vi "hReadChannels-UandP-2013.bak.vi"(0 "FPGA VI Reference In":refnum<k20>, 1 "SavGol side points":i32=10, 3 "Use Voltage or Power for AO?":bool, 4 "order polynomial":i32=2, 5 "Nsamples":u32=10000, 6 "error in":errorcluster, 8 "output cluster":T3, 9 "calculation settings":i32(slide) scale=0.0..3.0, 10 "variables cluster":T2, 11 "No. Of Samples to average":i32=10) -> (2 "Fehler":bool, 13 "AdjustedArray":sgl[][](array[numeric]), 18 "single channel voltage array":dbl[](array[numeric]), 19 "real time P_rad array":dbl[](array[numeric]), 20 "FPGA VI Reference Out":refnum<k20>, 22 "PowerArray":sgl[][](array[numeric]), 25 "RawArray":sgl[][](array[numeric]), 26 "error out":errorcluster)   [LabVIEW 2014]
doc: "startet das einlesen und führt dies bis n Samples aus\nHier mit FIFO und IRQ."
uses:
  <vilib>/Utility/error.llb/Error Cluster From Error Code.vi
  <vilib>/rvi/errors/niLvFpgaAdjustHostInterfaceError.vi
  <vilib>/RVI Host/nirviSupport.llb/nirviErrorClusterFromErrorCode.vi
  <vilib>/rvi/interface/nirviReadWriteControl/nirviReadWriteControl.xnode
  FPGA Bitfiles/W7XBolo2017_FPGATarget_fmain2014_DACRangeVoltage.lvbitx
  f_main_2014.vi
  <vilib>/rvi/interface/nirviMethod/nirviMethod.xnode
  NiFpgaLv.dll
  <vilib>/rvi/interface/nirviMethod/StockFPGA_InlinedMethodWaitForMultipleIRQ.vi
  <vilib>/FPGAPlugInAG/PCI-7813R/niLvFpga_WaitOnIrq_PCI-7813R.vi
  <vilib>/FPGAPlugInAG/PCI-7813R/niLvFpga_AcknowledgeIrq_PCI-7813R.vi
  <vilib>/FPGAPlugInAG/PCI-7813R/niLvFpga_ReadFifo_PCI-7813R.vi
  <vilib>/rvi/errors/niLvFpgaMergeErrorWithErrorCode.vi
panel:
  in  "Tab Control":T1(tab)
  out "16bit integer voltage sample":i16[](array[numeric])
  out "RTPRad voltage factor":dbl
  out "Timed Out":bool
  out "STOP?":bool
  out "Elements Remaining":u32
  out "single channel voltage":sgl
  out "single channel voltage * factor":dbl
  out "empty sample array":dbl[](array[numeric])
  out "Nsamples array":i64[](array[numeric])
  out "sample":i32
  out "new level of override":i32
  out "sate":string
  out "last U sample":sgl[](array[numeric])
  out "current P_rad [MW]":dbl
  out "rt prad average array":dbl[][](array[numeric])
  out "elec. channel selected":i64
  out "element of channel\nand sample":sgl
  out "column":i32
  out "channel index":i32
  out "av/f_OT*volume/k_bolo/V_cam":dbl
  out "average":dbl
  out "sum":dbl
  out "av/f_OT*volume":dbl
  out "average/f_OT":sgl
  out "av/f_OT*volume/k_bolo":dbl
  in  "magic number":dbl=1.0
  out "current power":sgl[](array[numeric])
  out "prad av array":dbl[](array[numeric])
  out "index status":bool
  out "dU/dt":sgl[](array[numeric])
  out "channel number":i64
  out "RawScal":dbl[](array[numeric])
  out "Scale(mV)":sgl[](array[numeric])
  out "SumScal":dbl[](array[numeric])
  out "Tau/dt":dbl[](array[numeric])
  out "F_ch":dbl[](array[numeric])
  out "tau_fact":dbl[](array[numeric])
  out "kbolott_and_volume":dbl[][](array[numeric])
  out "samples to exclude":u32
  out "single channel number":i64
  out "channelNumber":i32
  out "channelSelection":i64[][](array[numeric])
  out "tau_M":dbl[](array[numeric])
  out "Offsets":dbl[](array[numeric])
  out "SampleTime":sgl
  out "voltage factor":dbl
  out "Scale(mV) transf.":sgl[](array[numeric])
  out "V_cam":dbl
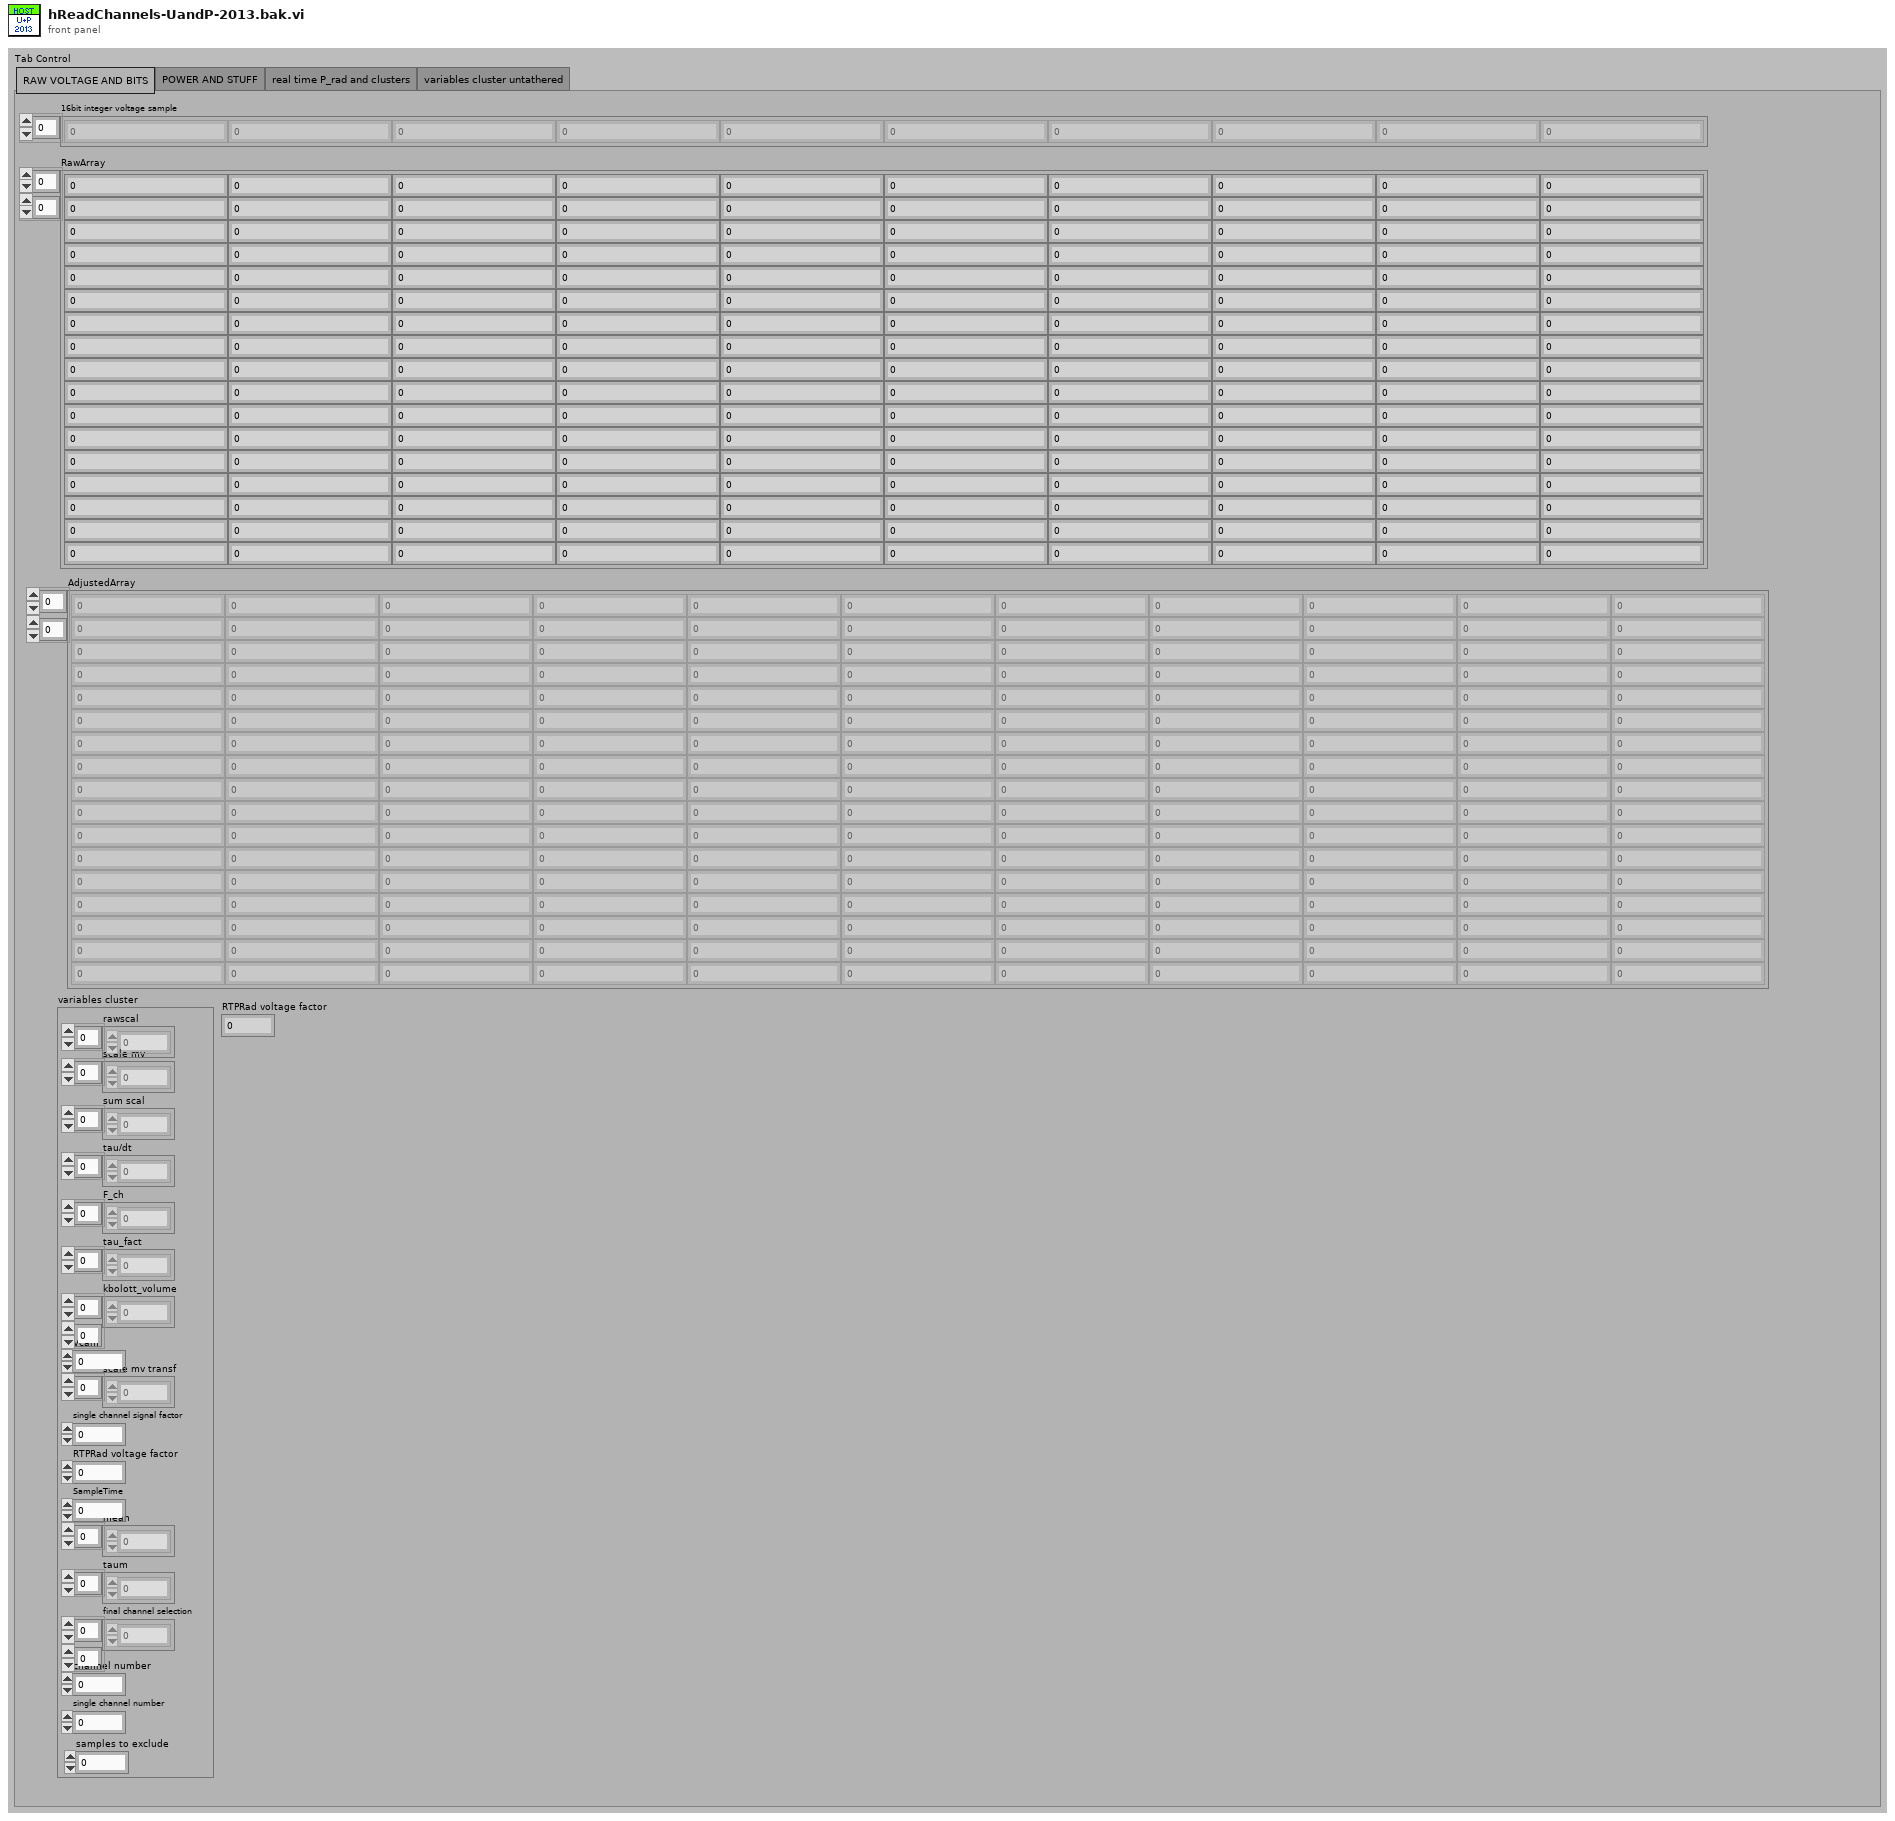
[diagram p1: front panel]
types:
  T1 = enum32{"RAW VOLTAGE AND BITS", "POWER AND STUFF", "real time P_rad and clusters", "variables cluster untathered"}
  T2 = cluster{"rawscal":dbl[], "scale mv":sgl[], "sum scal":dbl[], "tau/dt":dbl[], "F_ch":dbl[], "tau_fact":dbl[], "kbolott_volume":dbl[][], "Vcam":dbl, "scale mv transf":sgl[], "single channel signal factor":dbl, "RTPRad voltage factor":dbl, "SampleTime":sgl, "mean":dbl[], "taum":dbl[], "final channel selection":i64[][], "channel number":i32, "single channel number":i64, "samples to exclude":u32}
  T3 = cluster{"real time P_rad":refnum<vi>, "real time P_rad array":refnum<vi>, "single channel voltage":refnum<vi>, "single channel voltage array":refnum<vi>}
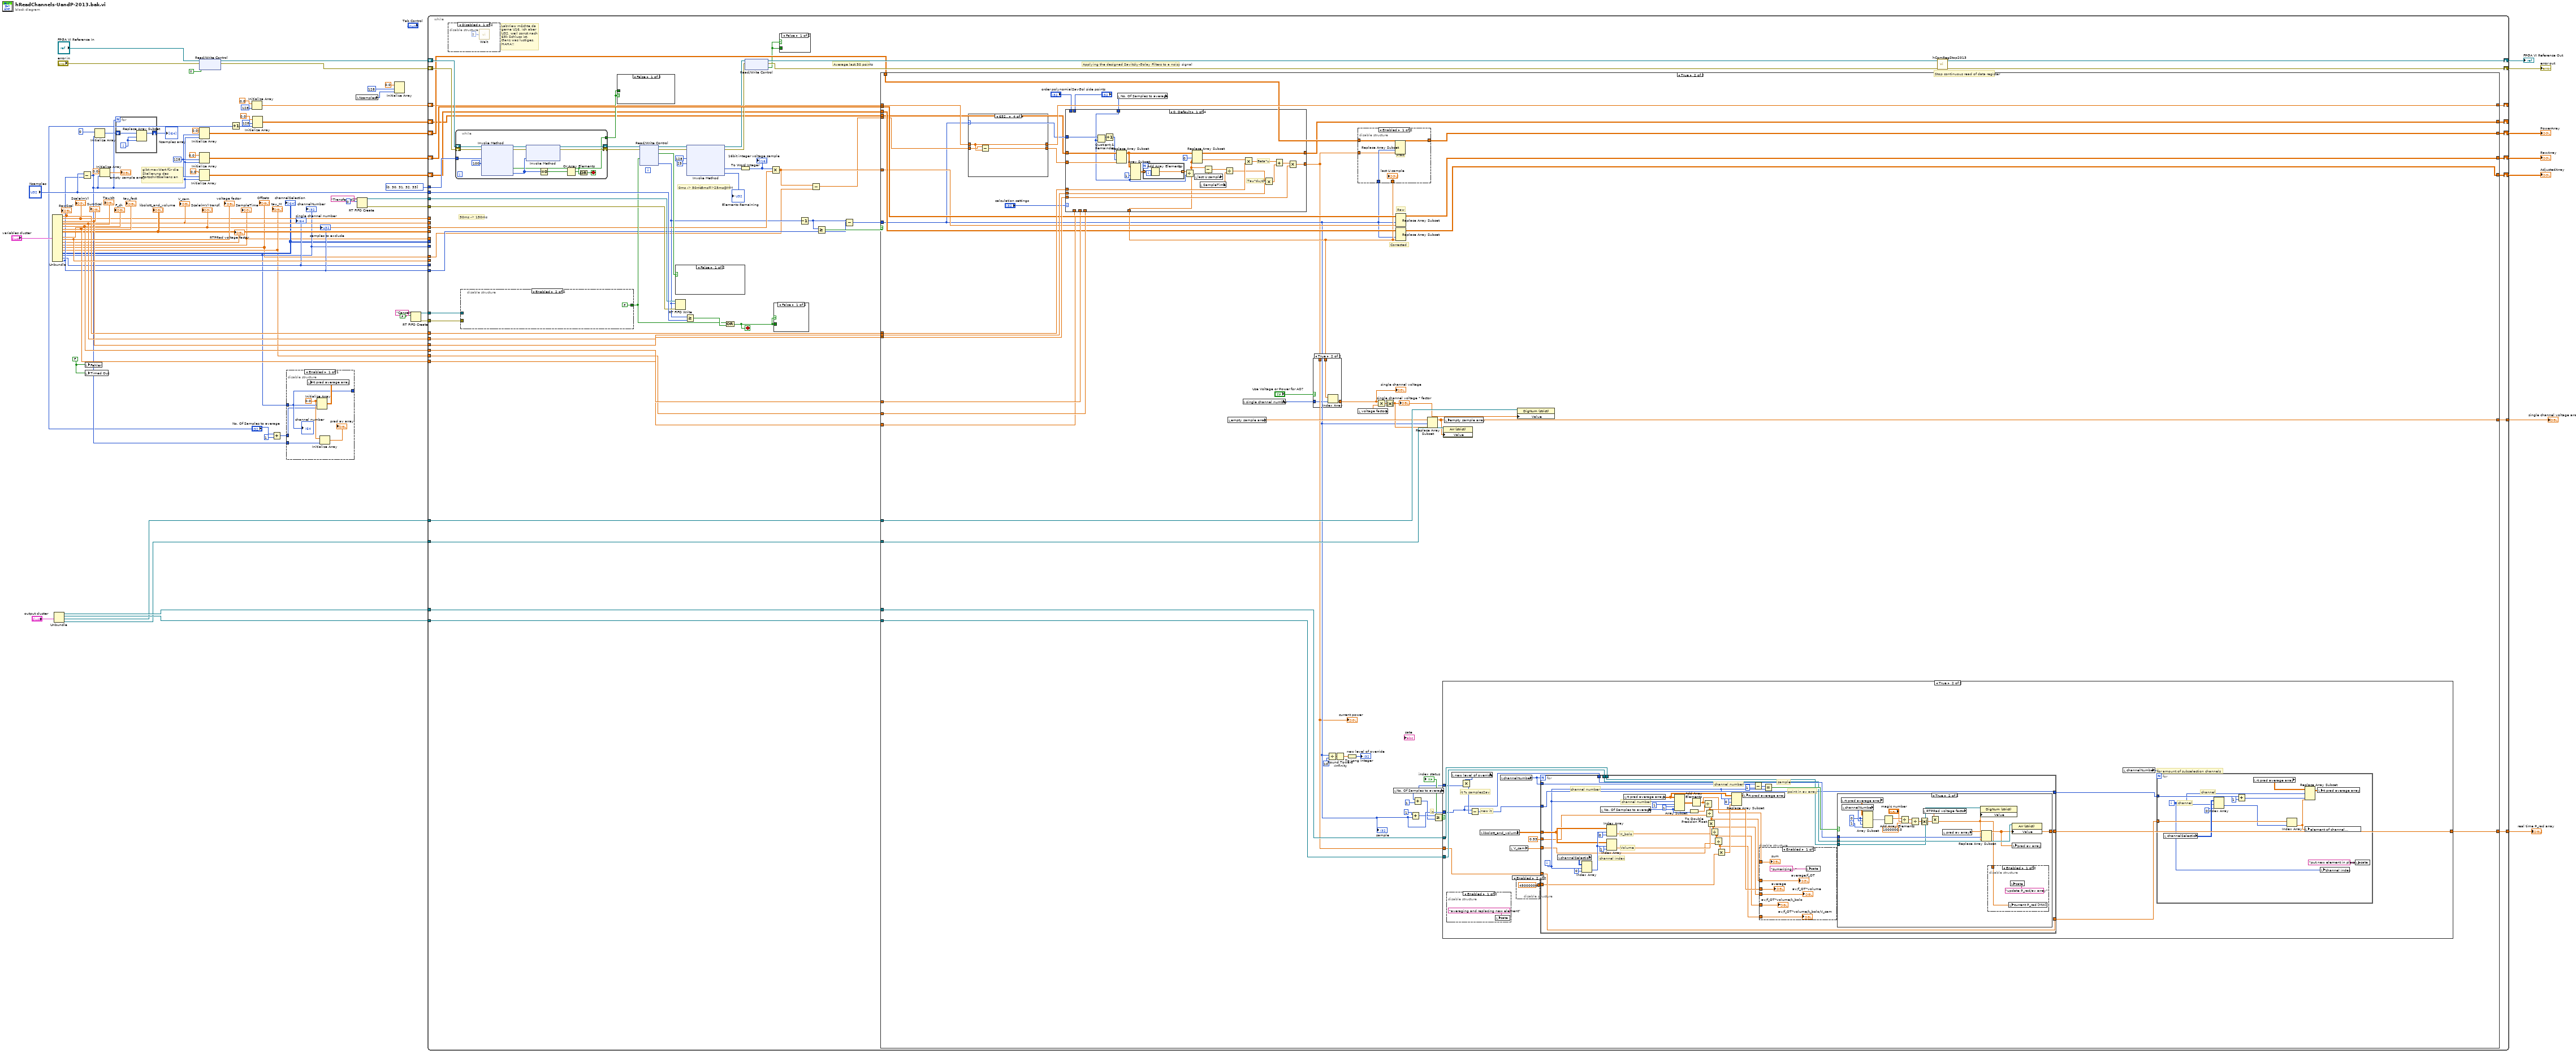
[diagram p0: block diagram]
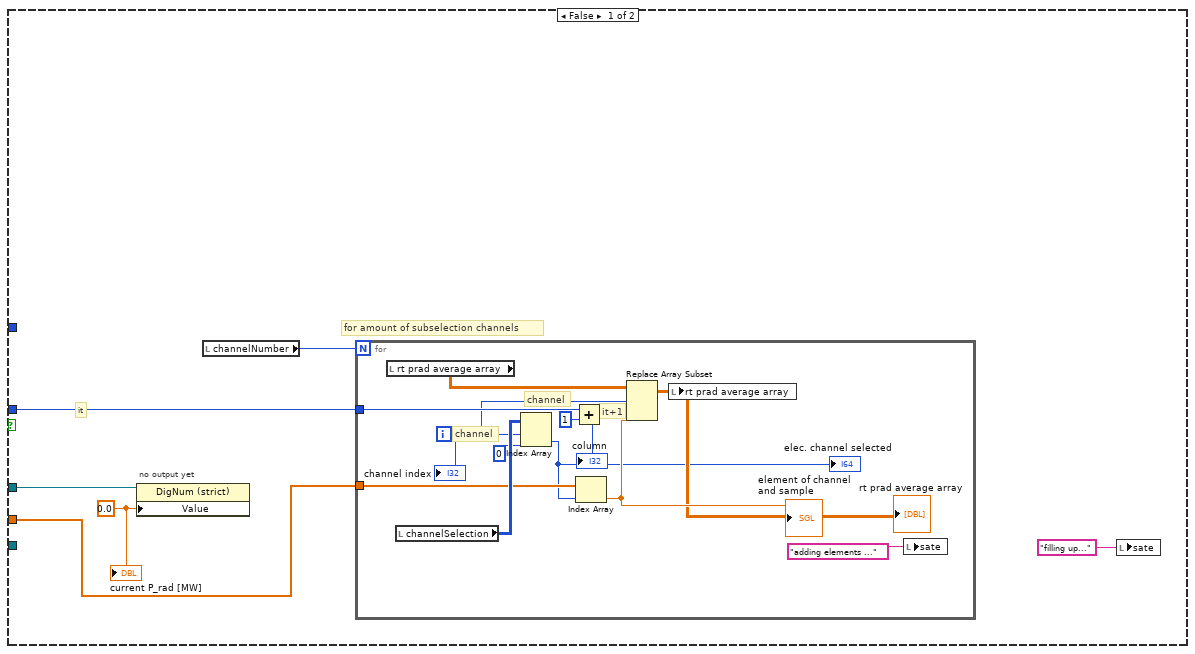
[diagram p3: hidden frame]
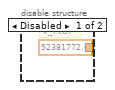
[diagram p4: hidden frame]
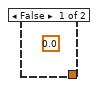
[diagram p7: hidden frame]
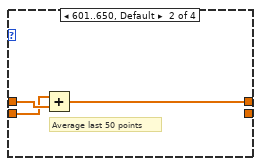
[diagram p10: hidden frame]
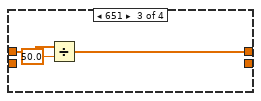
[diagram p11: hidden frame]
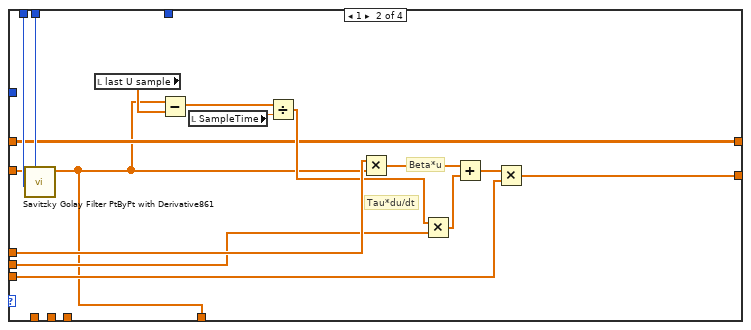
[diagram p12: hidden frame]
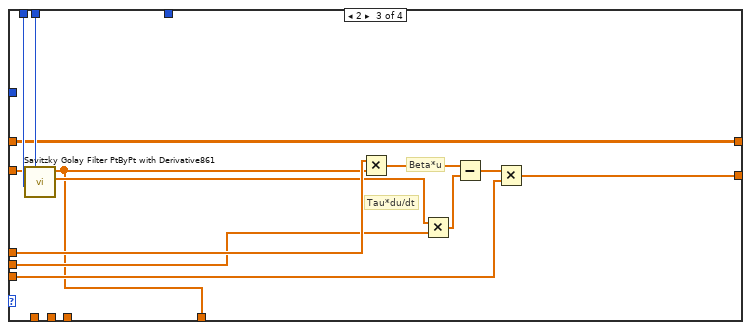
[diagram p13: hidden frame]
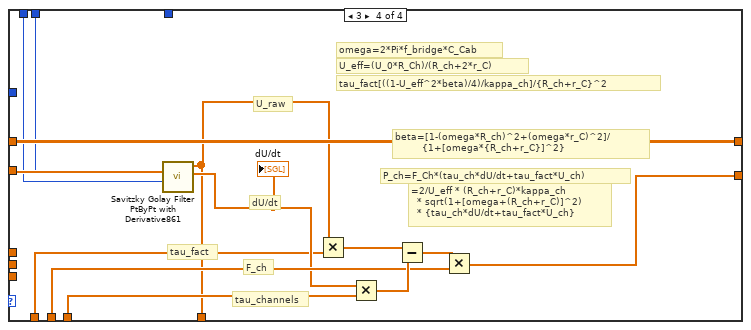
[diagram p14: hidden frame]
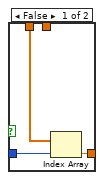
[diagram p15: hidden frame]
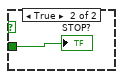
[diagram p17: hidden frame]
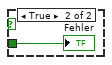
[diagram p18: hidden frame]
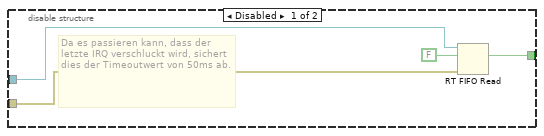
[diagram p19: hidden frame]
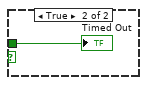
[diagram p20: hidden frame]
diagram:
  w44 = FALSE
  w19 = 128 ("dimension size")
  # "Stop continuous read of data register"
  # "gibt maxWert für die Skalierung des Fortschrittbalkens an"
  n1 = Unbundle("variables cluster") -> ("rawscal"=w35:dbl[], "scale mv"=w30:sgl[], "sum scal"=w36:dbl[], "tau/dt"=w34:dbl[], "F_ch"=w33:dbl[], "tau_fact"=w32:dbl[], "kbolott_volume"=w31:dbl[][], "Vcam"=w28:dbl, "scale mv transf"=w29:sgl[], "single channel signal factor"=w37:dbl, "RTPRad voltage factor"=→"RTPRad voltage factor":dbl, "SampleTime"=w8:sgl, "mean"=w9:dbl[], "taum"=w10:dbl[], "final channel selection"=w11:i64[][], "channel number"=w12:i32, "single channel number"=w13:i64, "samples to exclude"=w14:u32)
  "RawScal" <- w35
  "Scale(mV)" <- w30
  "SumScal" <- w36
  "Tau/dt" <- w34
  "F_ch" <- w33
  "tau_fact" <- w32
  "kbolott_and_volume" <- w31
  "V_cam" <- w28
  "Scale(mV) transf." <- w29
  "voltage factor" <- w37
  "SampleTime" <- w8
  "Offsets" <- w9
  "tau_M" <- w10
  "channelSelection" <- w11
  "channelNumber" <- w12
  "single channel number" <- w13
  "samples to exclude" <- w14
  n2 = Unbundle("output cluster") -> ("real time P_rad"=w39:refnum<vi>, "real time P_rad array"=w38:refnum<vi>, "single channel voltage"=w24:refnum<vi>, "single channel voltage array"=w23:refnum<vi>)
  n3 = Subtract(x="Nsamples", y=w14) -> (x-y=w18:u32)
  n4 = local write "Fehler"(w44) -> ()
  n5 = local write "Timed Out"(w44) -> ()
  n6 = Initialize Array(i64 0 ("element"), w18) -> (w46:i64[])
  n7 = Initialize Array(0.0 ("element"), w18) -> (→"empty sample array":dbl[])
  n8 = for {
    N: w18 -> [_]
    shift-right: [w76] -> w45
    shift-left: w46 -> [w78]
    i -> [w77]
    n9 = Replace Array Subset(array=w78, new element=w77, index=w77) -> (w76:i64[])
  }
  "Nsamples array" <- w45
  n10 = Initialize Array(sgl 0.0 ("element"), w19, w18) -> (w17:sgl[][])
  n11 = xnode "Read/Write Control"("FPGA VI Reference In"="FPGA VI Reference In", "error in"="error in", "ADCRead"=TRUE) -> ("FPGA VI Reference Out"=w57:refnum<k20>, "error out"=w56:errorcluster)
  n12 = Initialize Array(sgl 0.0 ("i"), w19, w18) -> (w66:sgl[][])
  n13 = Initialize Array(sgl 0.0, w19, w18) -> (w75:sgl[][])
  n14 = Increment(x="No. Of Samples to average") -> (x+1=w1:i32)
  n15 = Initialize Array(sgl 0.0 ("element"), 128 ("dimension size")) -> (w52:sgl[])
  n16 = Initialize Array(sgl 0.0 ("element"), 128 ("dimension size"), w1) -> (w3:sgl[][])
  n17 = Add(x="No. Of Samples to average", y=1) -> (x+y=w26:i32)
  n18 = disable-structure shown="Enabled" {
    disable-tunnel: w12 -> [w83]
    disable-tunnel: [w83] -> _
    disable-tunnel: w26 -> [w79]
    disable-tunnel: w18 -> [w80]
    frame Enabled {
      w82 = 0.0 ("element")
      n19 = Initialize Array(w82, w83, w79) -> (w84:dbl[][])
      n20 = local write "rt prad average array"(w84) -> ()
      n21 = Initialize Array(w82, w80) -> (→"prad av array":dbl[])
      "channel number" <- w83
    }
  }
  n22 = local read "Nsamples"() -> (w41:u32)
  n23 = RT FIFO Create(0:"Transferred1" ("name (unnamed)"), 1:u32 0) -> (8:w72:refnum<k33>, 11:w71:errorcluster)  [unwired: 2 in, 5 out]
  n24 = Initialize Array(sgl 0.0 ("element"), 128 ("dimension size"), w41) -> ()  [unwired: 1 out]
  n25 = RT FIFO Create(0:"Cancel" ("name (unnamed)"), 1:FALSE) -> (8:w69:refnum<k33>, 11:w68:errorcluster)  [unwired: 2 in, 5 out]
  n26 = while {
    tunnel: "Nsamples" -> [w137]
    shift-right: [w105] -> w15
    shift-left: w75 -> [w126]
    shift-right: [w138] -> w65
    shift-left: w57 -> [w141]
    shift-right: [w139] -> w64
    shift-left: w56 -> [w140]
    tunnel: w72 -> [w136]
    tunnel: w71 -> [w135]
    tunnel: w69 -> [w133]
    tunnel: w68 -> [w132]
    shift-right: [w130] -> w60
    shift-left: w66 -> [w131]
    tunnel: w29 -> [w125]
    tunnel: w34 -> [w122]
    tunnel: w36 -> [w124]
    tunnel: w35 -> [w123]
    shift-right: [w115] -> _
    shift-left: w52 -> [w91]
    tunnel: i32[] [0, 30, 31, 32, 33] -> [w110]
    tunnel: w23 -> [w107]
    tunnel: w24 -> [w106]
    tunnel: w13 -> [_]
    tunnel: w37 -> [_]
    tunnel: w9 -> [w87]
    tunnel: w14 -> [w88]
    tunnel: w39 -> [w102]
    tunnel: w38 -> [w97]
    tunnel: w33 -> [w101]
    tunnel: w32 -> [w100]
    tunnel: w30 -> [_]
    tunnel: w31 -> [_]
    tunnel: w8 -> [_]
    tunnel: w10 -> [w99]
    tunnel: w11 -> [_]
    tunnel: w12 -> [_]
    tunnel: w28 -> [_]
    tunnel: [w96] -> w22
    tunnel: [w95] -> w21
    shift-right: [w93] -> w16
    shift-left: w17 -> [w94]
    shift-right: [w85] -> _
    shift-left: w3 -> [w86]
    stop <- w111 stop-if-true
    # "Average last 50 points"
    # "Applying the designed Savitzky-Golay Filters to a noisy signal"
    # "LabView möchte da gerne U16, ich aber U32, weil sonst nach 65k Schluss ist. \nGanz was lustiges, HAHA!!"
    # "5ms=>25ms@MM"
    # "0ms -> 50ms"
    # "50ms -> 150ms"
    n27 = disable-structure shown="Disabled" {
      frame Disabled {
        n28 = call "Wait"("Count(uSec)"=u32 5) -> ()  [unwired: 1 out]
      }
      frame Enabled {
      }
    }
    n29 = while {
      tunnel: [w404] -> w114
      shift-right: [w406] -> w108
      shift-left: w141 -> [w413]
      shift-right: [w405] -> w109
      shift-left: w140 -> [w412]
      tunnel: w110 -> [w410]
      stop <- w403 stop-if-true
      n30 = xnode "Invoke Method"("FPGA VI Reference In"=w413, "error in"=w412, "IRQ Number(s)"=w410, "Timeout (ms)"=100) -> ("FPGA VI Reference Out"=w407:refnum<k20>, "error out"=w408:errorcluster, "Timed Out"=w404:bool, "IRQ(s) Asserted"=w409:i32[])
      n31 = xnode "Invoke Method"("FPGA VI Reference In"=w407, "error in"=w408, "IRQ Number(s)"=w409) -> ("FPGA VI Reference Out"=w406:refnum<k20>, "error out"=w405:errorcluster)
      n32 = Equal To 0?(x=w409) -> (x = 0?=w402:bool[])
      n33 = Or Array Elements(Boolean array=w402) -> (logical OR=w401:bool)
      n34 = Or(x=w401, y=w404) -> (x .or. y?=w403:bool)
    }
    n35 = disable-structure shown="Enabled" {
      disable-tunnel: [w419 FALSE] -> w134
      disable-tunnel: w133 -> [w418 _]
      disable-tunnel: w132 -> [w417 _]
      frame Disabled {
        # "Da es passieren kann, dass der letzte IRQ verschluckt wird, sichert dies der Timeoutwert von 50ms ab."
        n36 = RT FIFO Read(0:w418, 1:FALSE ("element"), 3:w417) -> (9:w419:bool)  [unwired: 5 out]
      }
      frame Enabled {
      }
    }
    n37 = case shown="False" w114 {
      tunnel: w114 -> [_ w421]
      frame False {
      }
      frame True {
        "Timed Out" <- w421
      }
    }
    n38 = xnode "Read/Write Control"("FPGA VI Reference In"=w108, "error in"=w109, "cancel"=w134) -> ("FPGA VI Reference Out"=w128:refnum<k20>, "error out"=w127:errorcluster, "Timeout"=w129:bool, "ScanID"=w92:u32)
    n39 = case shown="False" w129 {
      selector: w129 -> [_ w423]
      frame False {
      }
      frame True {
        n40 = local write "Fehler"(w423) -> ()
      }
    }
    n41 = RT FIFO Write(0:w136, 1:w92, 3:w135) -> ()  [unwired: 1 in, 5 out]
    n42 = Greater Or Equal?(x=w92, y=w137) -> (x >= y?=w142:bool)
    n43 = xnode ("Invoke Method")("FPGA VI Reference In"=w128, "error in"=w127, "Number of Elements"=u32 128, "Timeout (ms)"=25 ("Timeout")) -> ("FPGA VI Reference Out"=w117:refnum<k20>, "error out"=w116:errorcluster, "Data"=w119:u32[], "Elements Remaining"=→"Elements Remaining":u32)
    n44 = Compound Arithmetic op=OR(w134, w142) -> (w111:bool)
    n45 = To Word Integer(number=w119) -> (16bit integer=w118:i16[])
    "16bit integer voltage sample" <- w118
    n46 = xnode "Read/Write Control"("FPGA VI Reference In"=w117, "error in"=w116) -> ("FPGA VI Reference Out"=w138:refnum<k20>, "error out"=w139:errorcluster, "Fifo-Fehler"=w112:bool)
    n47 = Multiply(x=w118, y=w125) -> (x*y=w90:sgl[])
    n48 = case shown="False" w111 {
      tunnel: w111 -> [_ w414]
      frame False {
      }
      frame True {
        "STOP?" <- w414
      }
    }
    n49 = case shown="False" w112 {
      tunnel: w112 -> [_ w415]
      frame False {
      }
      frame True {
        "Fehler" <- w415
      }
    }
    n50 = Decrement(x=w92) -> (x-1=w103:u32)
    n51 = Subtract(x=w90, y=w87) -> (x-y=w89:dbl[])
    n52 = Greater Or Equal?(x=w103, y=w88) -> (x >= y?=w104:bool)
    n53 = Subtract(x=w103, y=w88) -> (x-y=w98:u32)
    n54 = case shown="True" w104 {
      tunnel: w131 -> [w146 w189]
      tunnel: [w146 w190] -> w130
      tunnel: w126 -> [w145 w188]
      tunnel: w124 -> [_ w196]
      tunnel: w123 -> [_ w195]
      tunnel: w122 -> [_ w194]
      tunnel: [w147 w193] -> w115
      tunnel: w91 -> [w147 w167]
      tunnel: w90 -> [_ w166]
      tunnel: w107 -> [_ w192]
      tunnel: w106 -> [_ w191]
      tunnel: [w145 w187] -> w105
      tunnel: w98 -> [_ w158]
      tunnel: w102 -> [_ w183]
      tunnel: w97 -> [_ w182]
      tunnel: w101 -> [_ w186]
      tunnel: w100 -> [_ w184]
      tunnel: w99 -> [_ w185]
      tunnel: [_ w172] -> w96
      tunnel: [_ w171] -> w95
      tunnel: w94 -> [w144 w169]
      tunnel: [w144 w168] -> w93
      tunnel: w89 -> [_ w165]
      tunnel: w86 -> [w143 w157]
      tunnel: [w143 w154] -> w85
      frame False {
      }
      frame True {
        # "it"
        # "Corrected"
        # "Raw"
        n55 = case shown="652.." w158 {
          tunnel: w165 -> [_ w312 _ w320]
          tunnel: [w311 w314 w315 w319] -> w193
          tunnel: w167 -> [w311 w313 w317 w319]
          tunnel: [_ _ _ w318] -> w156
          frame 0..600 {
          }
          frame 601..650, Default {
            # "Average last 50 points"
            n56 = Add(x=w312, y=w313) -> (x+y=w314:dbl[])
          }
          frame 651 {
            n57 = Divide(x=w317, y=sgl 50.0) -> (x/y=w315:dbl[])
          }
          frame 652.. {
            n58 = Subtract(x=w320, y=w319) -> (x-y=w318:dbl[])
          }
        }
        n59 = local read "No. Of Samples to average"() -> (w161:i32)
        n60 = case shown="0, Default" "calculation settings" {
          tunnel: w196 -> [w344 w362 w375 _]
          tunnel: w195 -> [w343 w361 w374 _]
          tunnel: w194 -> [w342 w360 w373 _]
          tunnel: [w341 w359 w372 w381] -> w155
          tunnel: "SavGol side points" -> [_ w358 w371 w378]
          tunnel: "order polynomial" -> [_ w357 w370 w377]
          tunnel: w156 -> [w340 w356 w369 w379]
          tunnel: w158 -> [w339 _ _ _]
          tunnel: w157 -> [w338 w348 w364 w380]
          tunnel: [w321 w348 w364 w380] -> w154
          tunnel: w185 -> [_ _ _ w385]
          tunnel: w186 -> [_ _ _ w384]
          tunnel: w184 -> [_ _ _ w382]
          tunnel: w161 -> [w323 _ _ _]
          tunnel: [w322 w347 w363 w376] -> w159
          frame 0, Default {
            # "Beta*u"
            # "Tau*du/dt"
            n61 = Quotient & Remainder(x=w339, y=w323) -> (x-y*floor(x/y)=w336:u32)  [unwired: 1 out]
            n62 = Increment(x=w336) -> (x+1=w337:u32)
            n63 = Replace Array Subset(array=w338, new element=w340, index (col)=w337) -> (w332:sgl[][])  [unwired: 1 in]
            n64 = Array Subset(array=w332, index (col)=1 ("index"), length (col)=w323) -> (w334:sgl[][])  [unwired: 2 in]
            n65 = for {
              tunnel: w334 -> [w346] mode=indexing
              tunnel: [w345] -> w333 mode=indexing
              n66 = Add Array Elements(numeric array=w346) -> (sum=w345:sgl)
            }
            n67 = Divide(x=w333, y=w323) -> (x/y=w322:sgl[])
            n68 = Replace Array Subset(array=w332, new element=w322, index (col)=0 ("index")) -> (w321:sgl[][])  [unwired: 1 in]
            n69 = local read "last U sample"() -> (w330:sgl[])
            n70 = local read "SampleTime"() -> (w328:sgl)
            n71 = Subtract(x=w322, y=w330) -> (x-y=w329:sgl[])
            n72 = Divide(x=w329, y=w328) -> (x/y=w324:sgl[])
            n73 = Multiply(x=w322, y=w343) -> (x*y=w327:dbl[])
            n74 = Multiply(x=w324, y=w342) -> (x*y=w325:dbl[])
            n75 = Add(x=w327, y=w325) -> (x+y=w326:dbl[])
            n76 = Multiply(x=w326, y=w344) -> (x*y=w341:dbl[])
          }
          frame 1 {
            # "Beta*u"
            # "Tau*du/dt"
            n77 = call "Savitzky Golay Filter PtByPt with Derivative861.vi"("order polynomial"=w357, "side points"=w358, "x"=w356) -> ("Filtered x"=w347:dbl[])  [unwired: 1 in, 7 out]
            n78 = local read "last U sample"() -> (w350:sgl[])
            n79 = Subtract(x=w347, y=w350) -> (x-y=w351:dbl[])
            n80 = local read "SampleTime"() -> (w349:sgl)
            n81 = Divide(x=w351, y=w349) -> (x/y=w353:dbl[])
            n82 = Multiply(x=w361, y=w347) -> (x*y=w355:dbl[])
            n83 = Multiply(x=w353, y=w360) -> (x*y=w352:dbl[])
            n84 = Add(x=w355, y=w352) -> (x+y=w354:dbl[])
            n85 = Multiply(x=w354, y=w362) -> (x*y=w359:dbl[])
          }
          frame 2 {
            # "Beta*u"
            # "Tau*du/dt"
            n86 = call "Savitzky Golay Filter PtByPt with Derivative861.vi"("order polynomial"=w370, "side points"=w371, "x"=w369) -> ("Filtered Derivative"=w365:dbl[], "Filtered x"=w363:dbl[])  [unwired: 1 in, 6 out]
            n87 = Multiply(x=w374, y=w363) -> (x*y=w368:dbl[])
            n88 = Multiply(x=w365, y=w373) -> (x*y=w366:dbl[])
            n89 = Subtract(x=w368, y=w366) -> (x-y=w367:dbl[])
            n90 = Multiply(x=w367, y=w375) -> (x*y=w372:dbl[])
          }
          frame 3 {
            # "beta=[1-(omega*R_ch)^2+(omega*r_C)^2]/\n         {1+[omega*{R_ch+r_C}]^2}"
            # "tau_fact[((1-U_eff^2*beta)/4)/kappa_ch]/{R_ch+r_C}^2"
            # "U_eff=(U_0*R_Ch)/(R_ch+2*r_C)"
            # "omega=2*Pi*f_bridge*C_Cab"
            # "=2/U_eff * (R_ch+r_C)*kappa_ch\n  * sqrt(1+[omega+(R_ch+r_C)]^2)\n  * {tau_ch*dU/dt+tau_fact*U_ch}"
            # "P_ch=F_Ch*(tau_ch*dU/dt+tau_fact*U_ch)"
            # "tau_channels"
            # "F_ch"
            # "tau_fact"
            # "U_raw"
            # "dU/dt"
            n91 = call "Savitzky Golay Filter PtByPt with Derivative861.vi"("order polynomial"=w377, "side points"=w378, "x"=w379) -> ("Filtered Derivative"=w383:dbl[], "Filtered x"=w376:dbl[])  [unwired: 1 in, 6 out]
            "dU/dt" <- w383
            n92 = Multiply(x=w376, y=w382) -> (x*y=w388:dbl[])
            n93 = Multiply(x=w383, y=w385) -> (x*y=w386:dbl[])
            n94 = Subtract(x=w388, y=w386) -> (x-y=w387:dbl[])
            n95 = Multiply(x=w387, y=w384) -> (x*y=w381:dbl[])
          }
        }
        "current power" <- w155
        n96 = local read "empty sample array"() -> (w179:dbl[])
        n97 = local read "single channel number"() -> (w181:i64)
        n98 = case shown="True" "Use Voltage or Power for AO?" {
          tunnel: w181 -> [w389 w394]
          tunnel: [w390 w393] -> w178
          tunnel: w159 -> [_ w392]
          tunnel: w155 -> [w391 _]
          frame False {
            n99 = Index Array(array=w391, index=w389) -> (element=w390:dbl)
          }
          frame True {
            n100 = Index Array(array=w392, index=w394) -> (element=w393:dbl)
          }
        }
        "single channel voltage" <- w178
        n101 = Divide(x=w158, y=10) -> (x/y=w174:dbl)
        n102 = Round Toward -Infinity(1:w174) -> (0:w175:dbl)
        n103 = To Long Integer(number=w175) -> (32bit integer=→"new level of override":i32)
        n104 = disable-structure shown="Enabled" {
          disable-tunnel: w189 -> [w399 w400]
          disable-tunnel: [w398 w400] -> w190
          disable-tunnel: w158 -> [w397 _]
          disable-tunnel: w155 -> [w396 _]
          disable-tunnel: w159 -> [w395 _]
          frame Enabled {
            # "Prad"
            n105 = Replace Array Subset(array=w399, new element=w396, index (col)=w397) -> (w398:sgl[][])  [unwired: 1 in]
            "last U sample" <- w395
          }
          frame Disabled {
          }
        }
        n106 = local read "voltage factor"() -> (w180:dbl)
        n107 = Multiply(x=w178, y=w180) -> (x*y=w177:dbl)
        n108 = Absolute Value(x=w177) -> (abs(x)=w164:dbl)
        "single channel voltage * factor" <- w164
        n109 = local read "No. Of Samples to average"() -> (w148:i32)
        n110 = Replace Array Subset(array=w188, new element=w166, index (col)=w158) -> (w187:sgl[][])  [unwired: 1 in]
        n111 = Replace Array Subset(array=w169, new element=w159, index (col)=w158) -> (w168:sgl[][])  [unwired: 1 in]
        n112 = Add(x=1, y=w158) -> (x+y=w151:u32)
        n113 = Add(x=w148, y=i64 1) -> (x+y=w149:i64)
        n114 = Replace Array Subset(array=w179, new element=w164, index=w158) -> (w171:dbl[])
        n115 = Greater Or Equal?(x=w151, y=w149) -> (x >= y?=w153:bool)
        "index status" <- w153
        n116 = case shown="True" w153 {
          tunnel: w158 -> [w198 w217]
          tunnel: w183 -> [w201 w219]
          tunnel: w182 -> [_ w220]
          tunnel: w155 -> [w199 w218]
          tunnel: w148 -> [_ w216]
          tunnel: [_ w215] -> w172
          frame False {
            w200 = 0.0 ("Value")
            # "it"
            # "for amount of subselection channels"
            # "no output yet"
            n117 = property class="DigNum (strict)"(reference=w201, "Value"=w200) -> ()  [unwired: 1 in, 2 out]
            n118 = local read "channelNumber"() -> (w202:i32)
            n119 = for {
              N: w202 -> [_]
              tunnel: w198 -> [w210]
              tunnel: w199 -> [w208]
              i -> [w205]
              # "channel"
              # "channel"
              # "it+1"
              n120 = local read "rt prad average array"() -> (w209:dbl[][])
              n121 = local read "channelSelection"() -> (w214:i64[][])
              n122 = Index Array(array=w214, index (row)=w205, index (col)=0 ("disabled index (col)")) -> (element=w204:i64)
              "elec. channel selected" <- w204
              n123 = Add(x=w210, y=1) -> (x+y=w211:u32)
              "column" <- w211
              n124 = Index Array(array=w208, index=w204) -> (element=w207:dbl)
              "element of channel\nand sample" <- w207
              n125 = Replace Array Subset(array=w209, new element=w207, index (row)=w205, index (col)=w211) -> (w206:dbl[][])
              "rt prad average array" <- w206
              n126 = local write "rt prad average array"(w206) -> ()
              n127 = local write "sate"("adding elements ...") -> ()
              "channel index" <- w205
            }
            n128 = local write "sate"("filling up...") -> ()
            "current P_rad [MW]" <- w200
          }
          frame True {
            # "new it"
            # "it % samples2av"
            # "for amount of subselection channels"
            n129 = disable-structure shown="Enabled" {
              frame Enabled {
                n130 = local write "sate"("averaging and replacing new element") -> ()
              }
              frame Disabled {
              }
            }
            n131 = local read "new level of override"() -> (w230:i32)
            n132 = Multiply(x=w230, y=w216) -> (x*y=w229:i32)
            n133 = Subtract(x=w217, y=w229) -> (x-y=w227:u32)
            n134 = local read "kbolott_and_volume"() -> (w228:dbl[][])
            n135 = local read "channelNumber"() -> (w222:i32)
            n136 = local read "V_cam"() -> (w224:dbl)
            n137 = disable-structure shown="Enabled" {
              disable-tunnel: [52381772.0 45000000.0] -> w226
              frame Disabled {
                # "V_Ptor"
              }
              frame Enabled {
              }
            }
            n138 = for {
              N: w222 -> [_]
              tunnel: w228 -> [w266]
              tunnel: [w271] -> w223
              tunnel: w218 -> [w271]
              tunnel: [w251] -> w221
              tunnel: w227 -> [w251]
              tunnel: w226 -> [w245]
              tunnel: 0.53 -> [w249]
              tunnel: w224 -> [w246]
              tunnel: w222 -> [w252]
              tunnel: w217 -> [w257]
              tunnel: w220 -> [w256]
              tunnel: w219 -> [w253]
              tunnel: [w235] -> w215
              i -> [w250]
              # "channel number"
              # "channel number"
              # "point in av array"
              # "sample"
              # "channel number"
              # "K_bolo"
              # "Volume"
              # "channel index"
              n139 = local read "channelSelection"() -> (w270:i64[][])
              n140 = Index Array(array=w270, index (row)=w250, index (col)=0 ("disabled index (col)")) -> (element=w267:i64)
              n141 = local read "No. Of Samples to average"() -> (w237:i32)
              n142 = Index Array(array=w266, index (row)=w267, index (col)=0 ("disabled index (col)")) -> (element=w247:dbl)
              n143 = Index Array(array=w266, index (row)=w267, index (col)=1 ("disabled index (col)")) -> (element=w248:dbl)
              n144 = local read "rt prad average array"() -> (w261:dbl[][])
              n145 = Array Subset(array=w261, index (row)=w250, length (row)=1, index (col)=1 ("index"), length (col)=w237) -> (w262:dbl[][])
              n146 = To Double Precision Float(number=w237) -> (double precision float=w236:dbl)
              n147 = Add Array Elements(numeric array=w262) -> (sum=w242:dbl)
              n148 = Divide(x=w242, y=w236) -> (x/y=w243:dbl)
              n149 = Divide(x=w243, y=w249) -> (x/y=w241:dbl)
              n150 = Multiply(x=w241, y=w248) -> (x*y=w240:dbl)
              n151 = Divide(x=w240, y=w247) -> (x/y=w239:dbl)
              n152 = Divide(x=w239, y=w246) -> (x/y=w238:dbl)
              n153 = Multiply(x=w238, y=w245) -> (x*y=w244:dbl)
              n154 = Replace Array Subset(array=w261, new element=w244, index (row)=w250, index (col)=0 ("disabled index (col)")) -> (w259:dbl[][])
              n155 = local write "rt prad average array"(w259) -> ()
              n156 = Subtract(x=w252, y=i64 1) -> (x-y=w255:i64)
              n157 = disable-structure shown="Enabled" {
                disable-tunnel: w243 -> [w277 _]
                disable-tunnel: w242 -> [w276 _]
                disable-tunnel: w241 -> [w275 _]
                disable-tunnel: w240 -> [w274 _]
                disable-tunnel: w239 -> [w273 _]
                disable-tunnel: w238 -> [w272 _]
                frame Enabled {
                  n158 = local write "sate"("sumarizing...") -> ()
                  "av/f_OT*volume/k_bolo" <- w273
                  "average/f_OT" <- w275
                  "av/f_OT*volume" <- w274
                  "sum" <- w276
                  "average" <- w277
                  "av/f_OT*volume/k_bolo/V_cam" <- w272
                }
                frame Disabled {
                }
              }
              n159 = Equal?(x=w255, y=w250) -> (x = y?=w258:bool)
              n160 = case shown="True" w258 {
                tunnel: w257 -> [_ w293]
                tunnel: w256 -> [_ w292]
                tunnel: w253 -> [_ w291]
                tunnel: [_ w282] -> w235
                frame False {
                  (unwired) 0.0
                }
                frame True {
                  w288 = 0 ("index")
                  n161 = local read "rt prad average array"() -> (w294:dbl[][])
                  n162 = local read "channelNumber"() -> (w289:i32)
                  n163 = Array Subset(array=w294, index (row)=w288, length (row)=w289, index (col)=w288, length (col)=1 ("index")) -> (w296:dbl[][])
                  n164 = Add Array Elements(numeric array=w296) -> (sum=w286:dbl)
                  n165 = Divide(x=w286, y="magic number") -> (x/y=w287:dbl)
                  n166 = Divide(x=w287, y=1000000.0) -> (x/y=w283:dbl)
                  n167 = Absolute Value(x=w283) -> (abs(x)=w281:dbl)
                  n168 = local read "RTPRad voltage factor"() -> (w279:dbl)
                  n169 = Multiply(x=w279, y=w281) -> (x*y=w280:dbl)
                  n170 = local read "prad av array"() -> (w284:dbl[])
                  n171 = property class="DigNum (strict)"(reference=w291, "Value"=w280) -> ()  [unwired: 1 in, 2 out]
                  n172 = Replace Array Subset(array=w284, new element=w280, index=w293) -> (w282:dbl[])
                  n173 = disable-structure shown="Enabled" {
                    disable-tunnel: w280 -> [w297 _]
                    frame Enabled {
                      n174 = local write "current P_rad [MW]"(w297) -> ()
                      n175 = local write "sate"("update P_rad/av array") -> ()
                    }
                    frame Disabled {
                    }
                  }
                  n176 = property class="Arr (strict)"(reference=w292, "Value"=w282) -> ()  [unwired: 1 in, 2 out]
                  n177 = local write "prad av array"(w282) -> ()
                }
              }
            }
            n178 = local read "channelNumber"() -> (w231:i32)
            n179 = for {
              N: w231 -> [_]
              tunnel: w221 -> [w306]
              tunnel: w223 -> [w304]
              i -> [w302]
              # "channel"
              # "channel"
              n180 = local read "channelSelection"() -> (w310:i64[][])
              n181 = Index Array(array=w310, index (row)=w302, index (col)=0 ("disabled index (col)")) -> (element=w300:i64)
              n182 = Add(x=w306, y=1) -> (x+y=w307:u32)
              n183 = local read "rt prad average array"() -> (w305:dbl[][])
              n184 = Index Array(array=w304, index=w300) -> (element=w301:dbl)
              n185 = local write "element of channel\nand sample"(w301) -> ()
              n186 = Replace Array Subset(array=w305, new element=w301, index (row)=w302, index (col)=w307) -> (w303:dbl[][])
              n187 = local write "rt prad average array"(w303) -> ()
              n188 = local write "channel index"(w302) -> ()
              n189 = local write "sate"("put new element in place") -> ()
            }
          }
        }
        n190 = property class="Arr (strict)"(reference=w192, "Value"=w171) -> ()  [unwired: 1 in, 2 out]
        n191 = local write "empty sample array"(w171) -> ()
        n192 = property class="DigNum (strict)"(reference=w191, "Value"=w164) -> ()  [unwired: 1 in, 2 out]
        "sample" <- w158
      }
    }
  }
  "RawArray" <- w15
  "PowerArray" <- w60
  "real time P_rad array" <- w22
  "single channel voltage array" <- w21
  "AdjustedArray" <- w16
  n193 = call "hComRegStop2013.vi"("error in"=w64, "FPGA VI Reference In"=w65) -> ("error out"=→"error out":errorcluster, "FPGA VI Reference Out"=→"FPGA VI Reference Out":refnum<k20>)  [unwired: 3 in, 1 out]
